vi "DefaultFromIni.vi"(8 "error in (no error)":errorcluster, 11 "SyncPlugin":refnum<class "PXI_MultiTrig.lvclass">) -> (0 "error out":errorcluster, 3 "SyncPlugin":refnum<class "PXI_MultiTrig.lvclass">)   [LabVIEW 2014, in "SyncPlugins.lvlib" / "PXI_MultiTrig.lvclass"]
uses:
  PXI_MultiTrig.lvclass
  Typedefs/TimeRefType.ctl
  Typedefs/clClocks.ctl
  Typedefs/clTrigger.ctl
  <userlib>/NIST/BaseClasses/BasePlugin_class/BasePlugin.lvclass/BasePlugin.ctl
  PXI_MultiTrig.lvclass/PXI_MultiTrig.ctl
  <userlib>/NIST/BaseClasses/BasePlugin_class/Accessors/Read PluginIniFilePath.vi
  Accessors/Write RefClkHandle.vi
  Accessors/Write TimingHandle.vi
  Accessors/Write Clocks.vi
  Accessors/Write Triggers.vi
  Accessors/Write TimeRefType.vi
  Accessors/Write SyncWindowsClock.vi
  SyncPluginBase/SyncPluginBase.lvclass
  <vilib>/Utility/config.llb/NI_LVConfig.lvlib
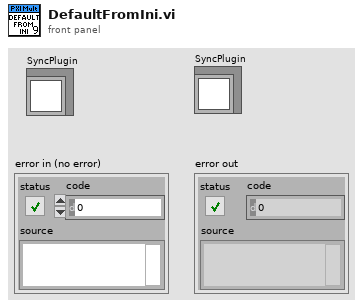
[diagram p1: front panel]
types:
  T1 = typedef "SyncPlugins.lvlib/PXI_MultiTrig.lvclass/clTrigger.ctl" = cluster{"Name":string, "DestTerm":string, "SrcTerm":string, "SyncClk":string, "Edge":i32, "Invert?":i32, "Initiated":bool, "Type":string, "TrigTime":bool}
  T2 = typedef "SyncPlugins.lvlib/PXI_MultiTrig.lvclass/clClocks.ctl" = cluster{"Name":string, "RefClk":string, "ClkTerminal":string, "Frequency":dbl, "DutyCycle":dbl, "ClkType":string, "Initiated":bool, "TrigTime":bool}
  T3 = typedef "SyncPlugins.lvlib/PXI_MultiTrig.lvclass/TimeRefType.ctl" = enum16{"1588", "Free Running", "GPS", "IRIG", "PPS"}
  T4 = typedef "NI_LVConfig.lvlib/Config Data RefNum.ctl" = refnum<k1>
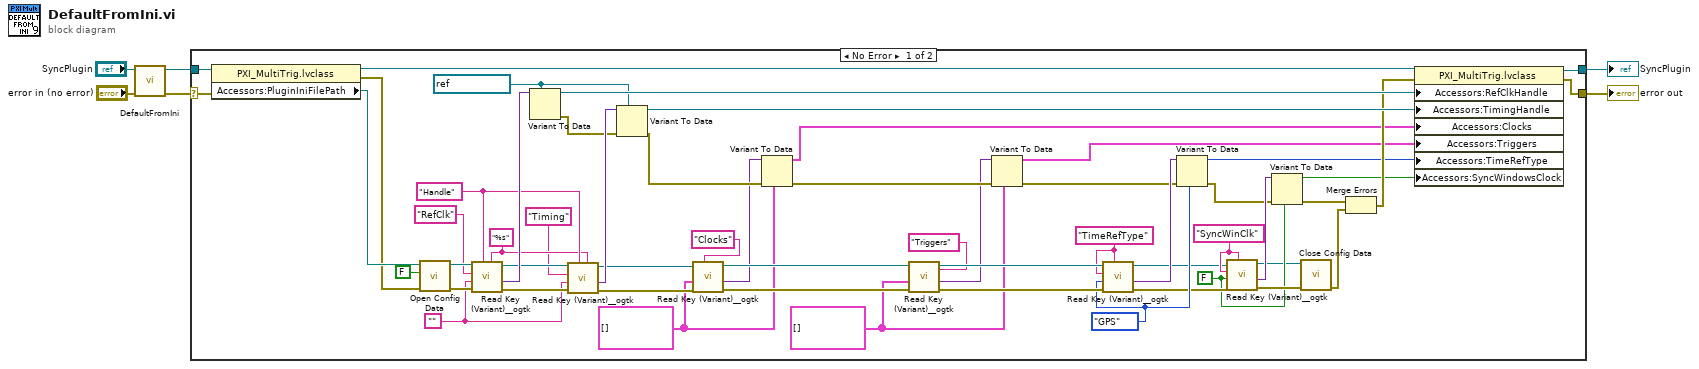
[diagram p0: block diagram]
diagram:
  n1 = call-parent "DefaultFromIni.vi"("error in (no error)"="error in (no error)", "SyncPlugin"="SyncPlugin") -> ("error out"=w4:errorcluster, "SyncPlugin"=w3:refnum<class "PXI_MultiTrig.lvclass">)  [unwired: 8 in]
  n2 = case shown="No Error" w4 {
    selector: w4 -> [w62 w63]
    tunnel: [w37 w64] -> w2
    tunnel: w3 -> [w61 w64]
    tunnel: [w38 w63] -> w1
    frame No Error {
      w9 = T1[] []
      w12 = T2[] []
      w21 = FALSE
      w22 = "SyncWinClk" ("section")
      w27 = TimeRefType."GPS" ("TimeRefType")
      w29 = "TimeRefType" ("section")
      w36 = ""
      w45 = refnum<k15> "PXI1Slot7" ("RefClkHandle")
      w49 = "Handle" ("section")
      w48 = "%s" ("format string (%;%f)")
      n3 = property class="PXI_MultiTrig.lvclass"(reference=w61, error in=w62) -> (reference out=w54:refnum<class "PXI_MultiTrig.lvclass">, error out=w59:errorcluster, "Accessors:PluginIniFilePath"=w60:path)
      n4 = call <vilib>:"Open Config Data.vi"("error in (no error)"=w59, "create file if necessary (T)"=FALSE, "configuration file path"=w60) -> ("error out"=w57:errorcluster, "refnum"=w56:T4)  [unwired: 6 in, 1 out]
      n5 = call <userlib>:"Read Key (Variant)__ogtk.vi"("format string (%;%f)"=w48, "section"=w49, "error in (no error)"=w57, "type"=w36, "key (optional)"="RefClk", "refnum"=w56) -> ("error out"=w50:errorcluster, "key-value"=w53:variant, "refnum out"=w51:T4)  [unwired: 2 in, 1 out]
      n6 = Variant To Data(type=w45, Variant=w53) -> (data=w52:refnum<k15>, error out=w43:errorcluster)  [unwired: 1 in]
      n7 = call <userlib>:"Read Key (Variant)__ogtk.vi"("format string (%;%f)"=w48, "section"=w49, "error in (no error)"=w50, "type"=w36, "key (optional)"="Timing", "refnum"=w51) -> ("error out"=w41:errorcluster, "key-value"=w46:variant, "refnum out"=w42:T4)  [unwired: 2 in, 1 out]
      n8 = Variant To Data(error in=w43, type=w45, Variant=w46) -> (data=w44:refnum<k15>, error out=w40:errorcluster)
      n9 = call <userlib>:"Read Key (Variant)__ogtk.vi"("section"="Clocks", "error in (no error)"=w41, "type"=w12, "refnum"=w42) -> ("error out"=w32:errorcluster, "key-value"=w14:variant, "refnum out"=w33:T4)  [unwired: 4 in, 1 out]
      n10 = Variant To Data(error in=w40, type=w12, Variant=w14) -> (data=w11:T2[], error out=w34:errorcluster)
      n11 = call <userlib>:"Read Key (Variant)__ogtk.vi"("section"="Triggers", "error in (no error)"=w32, "type"=w9, "refnum"=w33) -> ("error out"=w30:errorcluster, "key-value"=w10:variant, "refnum out"=w31:T4)  [unwired: 4 in, 1 out]
      n12 = Variant To Data(error in=w34, type=w9, Variant=w10) -> (data=w8:T1[], error out=w25:errorcluster)
      n13 = call <userlib>:"Read Key (Variant)__ogtk.vi"("section"=w29, "error in (no error)"=w30, "type"=w27, "key (optional)"=w29, "refnum"=w31) -> ("error out"=w23:errorcluster, "key-value"=w26:variant, "refnum out"=w16:T4)  [unwired: 3 in, 1 out]
      n14 = Variant To Data(error in=w25, type=w27, Variant=w26) -> (data=w28:T3, error out=w17:errorcluster)
      n15 = call <userlib>:"Read Key (Variant)__ogtk.vi"("section"=w22, "error in (no error)"=w23, "type"=w21, "key (optional)"=w22, "refnum"=w16) -> ("error out"=w24:errorcluster, "key-value"=w20:variant, "refnum out"=w15:T4)  [unwired: 3 in, 1 out]
      n16 = Variant To Data(error in=w17, type=w21, Variant=w20) -> (data=w18:bool, error out=w19:errorcluster)
      n17 = call <vilib>:"Close Config Data.vi"("error in (no error)"=w24, "refnum"=w15) -> ("error out"=w35:errorcluster)  [unwired: 8 in, 1 out]
      n18 = Merge Errors(w19, w35) -> (w39:errorcluster)
      n19 = property class="PXI_MultiTrig.lvclass"(reference=w54, error in=w39, "Accessors:RefClkHandle"=w52, "Accessors:TimingHandle"=w44, "Accessors:Clocks"=w11, "Accessors:Triggers"=w8, "Accessors:TimeRefType"=w28, "Accessors:SyncWindowsClock"=w18) -> (reference out=w37:refnum<class "PXI_MultiTrig.lvclass">, error out=w38:errorcluster)
    }
    frame Error {
    }
  }
  "SyncPlugin" <- w2
  "error out" <- w1
